vi "Data to Battery Status.vi"(1 "Data":u8[](array[numeric])) -> (0 "Battery Status":T1)   [LabVIEW 2016]
uses:
  Battery Status.ctl
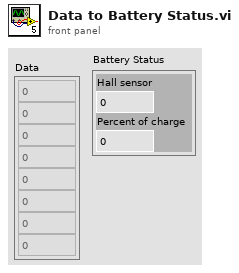
[diagram p1: front panel]
types:
  T1 = typedef "Battery Status.ctl" = cluster{"Hall sensor":i32, "Percent of charge":i16}
  T2 = cluster{"Data[0]":u8, "Data[1]":u8, "Data[2]":u8, "Data[3]":u8, "Data[4]":u8, "Data[5]":u8, "Data[6]":u8, "Data[7]":u8, "Data[8]":u8}
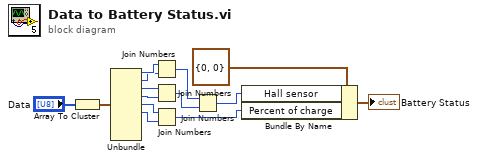
[diagram p0: block diagram]
diagram:
  n1 = Array To Cluster(array="Data") -> (cluster=w14:T2)
  n2 = Unbundle(w14) -> ("Data[0]"=w13:u8, "Data[1]"=w12:u8, "Data[2]"=w11:u8, "Data[3]"=w10:u8, "Data[4]"=w7:u8, "Data[5]"=w6:u8)  [unwired: 3 out]
  n3 = Join Numbers(hi=w13, lo=w12) -> ((hi.lo)=w9:u16)
  n4 = Join Numbers(hi=w11, lo=w10) -> ((hi.lo)=w8:u16)
  n5 = Join Numbers(hi=w7, lo=w6) -> ((hi.lo)=w2:u16)
  n6 = Join Numbers(hi=w9, lo=w8) -> ((hi.lo)=w3:u32)
  n7 = Bundle By Name(cluster=T1 {"Hall sensor"=0, "Percent of charge"=0} ("Battery Status"), "Hall sensor"=w3, "Percent of charge"=w2) -> (→"Battery Status":T1)
